vi "1DU8ToString.vi"(0 "Array":u8[](array[numeric]), 11 "Error in":errorcluster caption="Error in (no error)") -> (4 "String":string, 15 "Error out":errorcluster)   [LabVIEW 2017, in "GPString.lvlib"]
doc: "Converts <B>Array</B> to <B>String</B>.\n\nThis VI is inlined and it runs only if there is no error on <B>Error in</B>.\n\nSteen Schmidt\nGPower\n15/6 2016"
uses:
  GPString.lvlib
panel:
  # "Copyright © 2016\nGPower\nSee enclosed license file for terms and conditions"
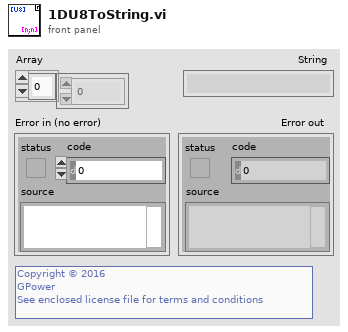
[diagram p1: front panel]
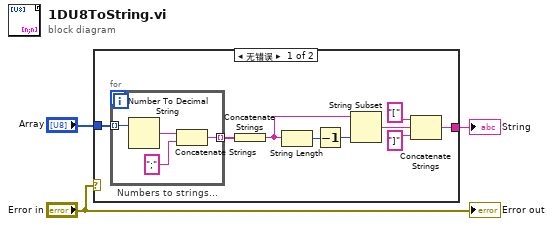
[diagram p0: block diagram]
diagram:
  n1 = case shown="无错误" "Error in" {
    tunnel: "Array" -> [w12 _]
    tunnel: [w8 _] -> w2
    frame No Error {
      n2 = for "Numbers to strings..." {
        tunnel: w12 -> [w15] mode=indexing
        tunnel: [w16] -> w11 mode=indexing
        n3 = Number To Decimal String(number=w15) -> (decimal integer string=w14:string)  [unwired: 1 in]
        n4 = Concatenate Strings(w14, ";" ("Secondary separator char")) -> (w16:string)
      }
      n5 = Concatenate Strings(w11) -> (w7:string)
      n6 = String Length(string=w7) -> (length=w5:i32)
      n7 = Decrement(x=w5) -> (x-1=w6:i32)
      n8 = String Subset(string=w7, length (rest)=w6) -> (substring=w4:string)  [unwired: 1 in]
      n9 = Concatenate Strings("[" ("substring"), w4, "]" ("substring")) -> (w8:string)
    }
    frame Error {
    }
  }
  "String" <- w2
  "Error out" <- "Error in"
